vi "SSC Digital PPMU Source Current.vi"(0 "Digital SSC in":T1[](array[typedef]), 5 "Current Level (A)":dbl, 7 "Current Level Range (A)":dbl format="%#_6p", 11 "error in":errorcluster) -> (4 "Digital SSC out":T1[](array[typedef]), 15 "error out":errorcluster)   [LabVIEW 2019]
doc: "Starts sourcing current from the PPMU on the specified pin(s) and pin group(s). This VI automatically selects the PPMU function. Changes to PPMU source settings do not take effect until you call this VI."
uses:
  SSC Digital.ctl
  <instrlib>/niDigital/niDigital.llb/niDigital Output Function.ctl
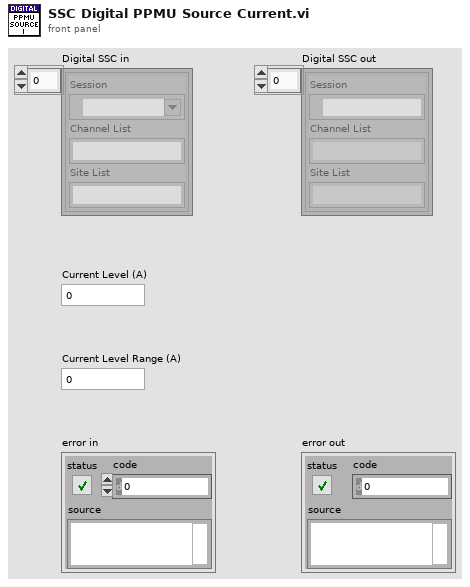
[diagram p1: front panel]
types:
  T1 = typedef "SSC Digital.ctl" = cluster{"Session":refnum<k15>, "Channel List":string, "Site List":string}
  T2 = typedef "niDigital Output Function.ctl" = i32
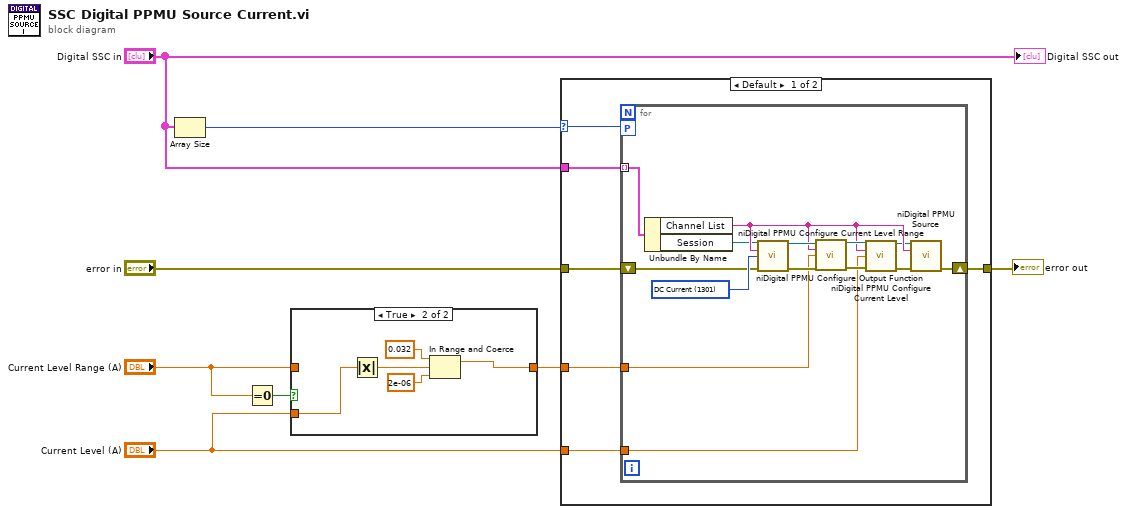
[diagram p0: block diagram]
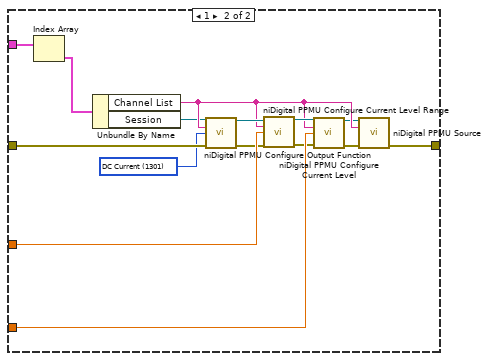
[diagram p2: hidden frame]
diagram:
  n1 = Array Size(array="Digital SSC in") -> (size(s)=w6:i32)
  n2 = Equal To 0?(x="Current Level Range (A)") -> (x = 0?=w4:bool)
  n3 = case shown="True" w4 {
    tunnel: [w9 w11] -> w3
    tunnel: "Current Level Range (A)" -> [w9 _]
    tunnel: "Current Level (A)" -> [_ w10]
    frame False {
    }
    frame True {
      n4 = Absolute Value(x=w10) -> (abs(x)=w14:dbl)
      n5 = In Range and Coerce(upper limit=0.032, x=w14, lower limit=2e-06 ("upper limit")) -> (coerced(x)=w11:dbl)  [unwired: 1 out]
    }
  }
  n6 = case shown="Default" w6 {
    selector: w6 -> [w18 _]
    tunnel: "error in" -> [w20 w49]
    tunnel: [w19 w48] -> w7
    tunnel: "Digital SSC in" -> [w17 w47]
    tunnel: w3 -> [w16 w46]
    tunnel: "Current Level (A)" -> [w15 w45]
    frame Default {
      n7 = for {
        tunnel: w15 -> [w29]
        workers-P: w18 -> [_]
        tunnel: w16 -> [w21]
        tunnel: w17 -> [w27] mode=indexing
        shift-right: [w28] -> w19
        shift-left: w20 -> [w23]
        w30 = T2 1301 items=["DC Voltage"=1300, "DC Current"=1301] ("output function")
        n8 = Unbundle By Name(w27) -> ("Channel List"=w26:string, "Session"=w22:refnum<k15>)
        n9 = call <instrlib>:"niDigital PPMU Configure Output Function.vi"("instrument handle"=w22, "channel list"=w26, "output function"=w30, "error in"=w23) -> ("instrument handle out"=w31:refnum<k15>, "error out"=w34:errorcluster)  [unwired: 10 in]
        n10 = call <instrlib>:"niDigital PPMU Configure Current Level Range.vi"("instrument handle"=w31, "channel list"=w26, "current level range (A)"=w21, "error in"=w34) -> ("instrument handle out"=w32:refnum<k15>, "error out"=w33:errorcluster)  [unwired: 10 in]
        n11 = call <instrlib>:"niDigital PPMU Configure Current Level.vi"("instrument handle"=w32, "channel list"=w26, "current level (A)"=w29, "error in"=w33) -> ("instrument handle out"=w25:refnum<k15>, "error out"=w24:errorcluster)  [unwired: 10 in]
        n12 = call <instrlib>:"niDigital PPMU Source.vi"("instrument handle"=w25, "channel list"=w26, "error in"=w24) -> ("error out"=w28:errorcluster)  [unwired: 11 in, 1 out]
      }
    }
    frame 1 {
      w40 = T2 1301 items=["DC Voltage"=1300, "DC Current"=1301] ("output function")
      n13 = Index Array(array=w47) -> (element=w35:T1)  [unwired: 1 in]
      n14 = Unbundle By Name(w35) -> ("Channel List"=w39:string, "Session"=w36:refnum<k15>)
      n15 = call <instrlib>:"niDigital PPMU Configure Output Function.vi"("instrument handle"=w36, "channel list"=w39, "output function"=w40, "error in"=w49) -> ("instrument handle out"=w41:refnum<k15>, "error out"=w44:errorcluster)  [unwired: 10 in]
      n16 = call <instrlib>:"niDigital PPMU Configure Current Level Range.vi"("instrument handle"=w41, "channel list"=w39, "current level range (A)"=w46, "error in"=w44) -> ("instrument handle out"=w42:refnum<k15>, "error out"=w43:errorcluster)  [unwired: 10 in]
      n17 = call <instrlib>:"niDigital PPMU Configure Current Level.vi"("instrument handle"=w42, "channel list"=w39, "current level (A)"=w45, "error in"=w43) -> ("instrument handle out"=w38:refnum<k15>, "error out"=w37:errorcluster)  [unwired: 10 in]
      n18 = call <instrlib>:"niDigital PPMU Source.vi"("instrument handle"=w38, "channel list"=w39, "error in"=w37) -> ("error out"=w48:errorcluster)  [unwired: 11 in, 1 out]
    }
  }
  "error out" <- w7
  "Digital SSC out" <- "Digital SSC in"
